vi "SwitchBoard_write.vi"(8 "error in":errorcluster, 10 "Buffer":string="MATRIX.SHORTALL", 11 "Handle":u32) -> (0 "error out":errorcluster, 2 "Bytes Written":u32, 3 "Handle":u32)   [LabVIEW 2016]
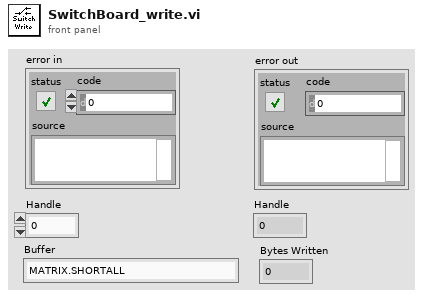
[diagram p1: front panel]
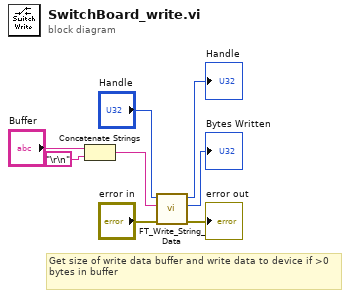
[diagram p0: block diagram]
diagram:
  # "Get size of write data buffer and write data to device if >0 bytes in buffer"
  n1 = Concatenate Strings("Buffer", "\r\n") -> (w5:string)
  n2 = call <instrlib>:"FT_Write_String_Data.vi"("error in"="error in", "Buffer"=w5, "Handle"="Handle") -> ("error out"=→"error out":errorcluster, "Bytes Written"=→"Bytes Written":u32, "Handle out"=→"Handle":u32)  [unwired: 6 in]
